vi "New UI Logger.vi"(6 "Level":T6, 7 "Logger Name":string, 8 "error in (no error)":errorcluster, 10 "General Options":T1={"Format"=[enum."Timestamp", enum."Message"], "Timestamp format"="%T", "Level Meaning"=enum."Standard", "Sorting"=enum."Add to Bottom"}, 11 "UI Options":T5={"Ctl Refnum"=refnum, "Delimiter"=" - "}) -> (0 "error out":errorcluster)   [LabVIEW 2020, in "Global_logger.lvlib"]
uses:
  Global_logger.lvlib
  Levels.ctl
  UI Options.ctl
  General Options.ctl
  Log Fields.ctl
  Level Meaning.ctl
  Sorting.ctl
  Logger Output.ctl
  Logger Type.ctl
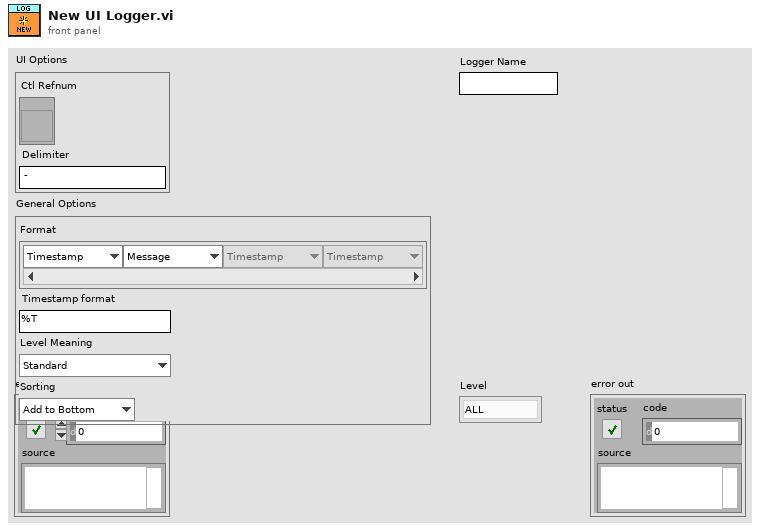
[diagram p1: front panel]
types:
  T1 = typedef "Global_logger.lvlib/General Options.ctl" = cluster{"Format":T2[], "Timestamp format":string, "Level Meaning":T3, "Sorting":T4}
  T2 = typedef "Global_logger.lvlib/Log Fields.ctl" = enum16{"Timestamp", "Level", "Message", "Source VI", "Source App", "Logger Name"}
  T3 = typedef "Global_logger.lvlib/Level Meaning.ctl" = enum16{"Standard", "Positive", "Exact"}
  T4 = typedef "Global_logger.lvlib/Sorting.ctl" = enum16{"Add to Bottom", "Add to Top"}
  T5 = typedef "Global_logger.lvlib/UI Options.ctl" = cluster{"Ctl Refnum":refnum<vi>, "Delimiter":string}
  T6 = typedef "Global_logger.lvlib/Levels.ctl" = enum16{"ALL", "TRACE", "DEBUG", "INFO", "WARN", "ERROR", "FATAL", "OFF"}
  T7 = typedef "Global_logger.lvlib/Logger Type.ctl" = enum16{"FILE", "UI"}
  T8 = typedef "Global_logger.lvlib/Logger Output.ctl" = cluster{"Level":T6, "Level Meaning":T3, "Sorting":T4, "Type":T7, "Filetype":string, "Filename":string, "Root path":path, "Max filesize (bytes)":i32, "Max age (days)":i32, "Ctl Refnum":refnum<vi>, "String Ctl Delimiter":string, "Format":T2[], "Timestamp format":string}
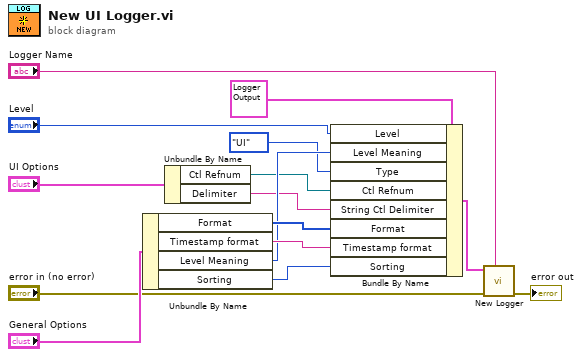
[diagram p0: block diagram]
diagram:
  n1 = Unbundle By Name("General Options") -> ("Format"=w11:T2[], "Timestamp format"=w10:string, "Level Meaning"=w9:T3, "Sorting"=w1:T4)
  n2 = Unbundle By Name("UI Options") -> ("Ctl Refnum"=w5:refnum<vi>, "Delimiter"=w2:string)
  n3 = Bundle By Name(cluster=T8 {"Level"=enum."ALL", "Level Meaning"=enum."Standard", "Sorting"=enum."Add to Bottom", "Type"=enum."FILE", "Filetype"="", "Filename"="", "Root path"=path "", "Max filesize (bytes)"=0, "Max age (days)"=0, "Ctl Refnum"=refnum, "String Ctl Delimiter"="", "Format"=[], "Timestamp format"=""} ("Logger Output"), "Level"="Level", "Level Meaning"=w9, "Type"=Logger_Type."UI", "Ctl Refnum"=w5, "String Ctl Delimiter"=w2, "Format"=w11, "Timestamp format"=w10, "Sorting"=w1) -> (w13:T8)
  n4 = call "New Logger.vi"("Logger Name"="Logger Name", "error in (no error)"="error in (no error)", "Logger Output in"=w13) -> ("error out"=→"error out":errorcluster)  [unwired: 8 in]
